vi "PLC_OutPut.vi"   [LabVIEW 2015]
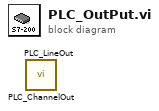
[diagram p0: block diagram]
diagram:
  n1 = call "PLC_ChannelOut.vi"() -> ()  [unwired: 6 in, 1 out]
  n2 = call "PLC_LineOut.vi"() -> ()  [unwired: 5 in, 2 out]
